vi "ELVIS III v1.0 DO Enqueue Data.vi"(7 "DO Block Channels FPGA Reference":T1, 8 "error in (no error)":errorcluster, 11 "DO Block Write Configuration":T2={"Wait Until Done?"=TRUE, "DO FIFO Clock Divisor"=1000, "Write Mode"=0, "DO (N Samples) Bank Data "=[]}) -> (0 "error out":errorcluster)   [LabVIEW 2021]
uses:
  <vilib>/myRIO/Common/Instrument Driver Framework/ELVIS III v1.0/DO Block/typedefs/ELVIS III DO Block Configuration.ctl
  <vilib>/myRIO/Common/Instrument Driver Framework/ELVIS III v1.0/DO Block/typedefs/ELVIS III DO Block Bank Data.ctl
  <vilib>/myRIO/Common/Instrument Driver Framework/ELVIS III v1.0/DO Block/typedefs/ELVIS III DO Block FPGA Reference.ctl
  <vilib>/rvi/errors/niLvFpgaAdjustHostInterfaceError.vi
  <vilib>/rvi/interface/nirviReadWriteControl/nirviReadWriteControl.xnode
  NiFpgaLv.dll
  <vilib>/rvi/interface/Simulation/niFpgaSimulationCallBeginRW.vi
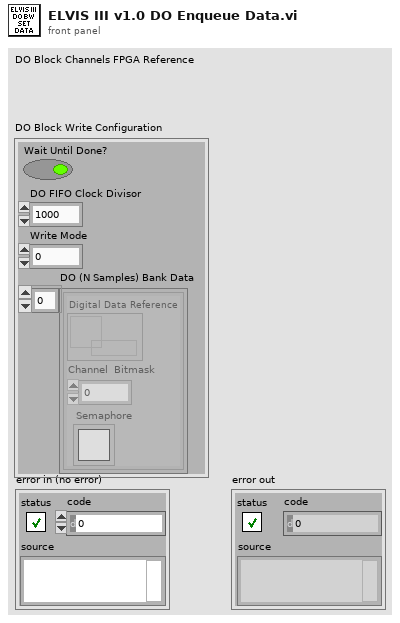
[diagram p1: front panel]
types:
  T1 = typedef "ELVIS III DO Block FPGA Reference.ctl" = refnum<k20>
  T2 = typedef "ELVIS III DO Block Configuration.ctl" = cluster{"Wait Until Done?":bool, "DO FIFO Clock Divisor":u16, "Write Mode":u8, "DO (N Samples) Bank Data ":T3[]}
  T3 = typedef "ELVIS III DO Block Bank Data.ctl" = cluster{"Digital Data Reference":refnum<data-value>, "Channel  Bitmask":fxp<+,20,20>, "Semaphore":T4}
  T4 = typedef "Semaphore RefNum" = refnum<k1>
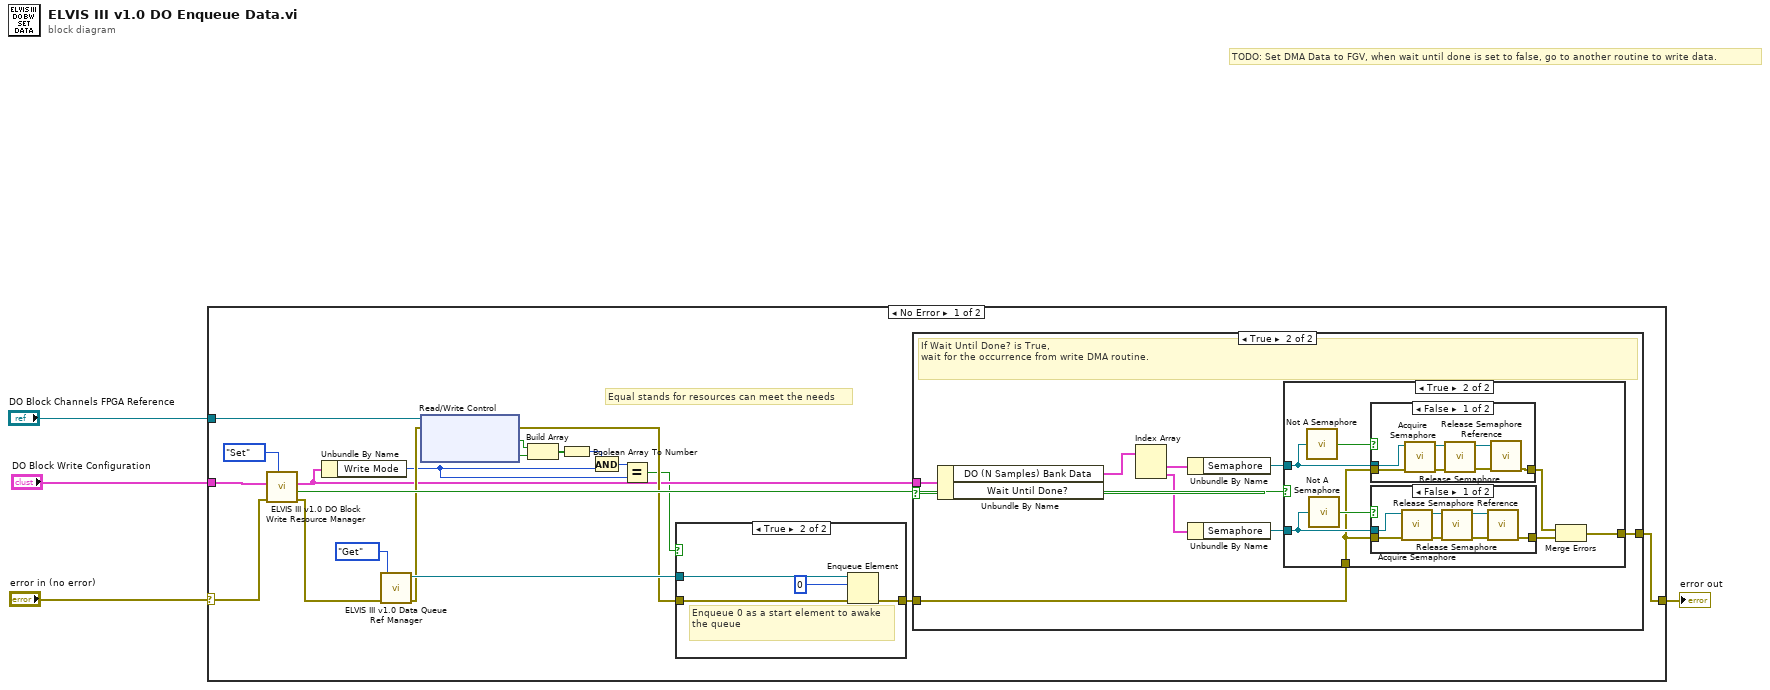
[diagram p0: block diagram]
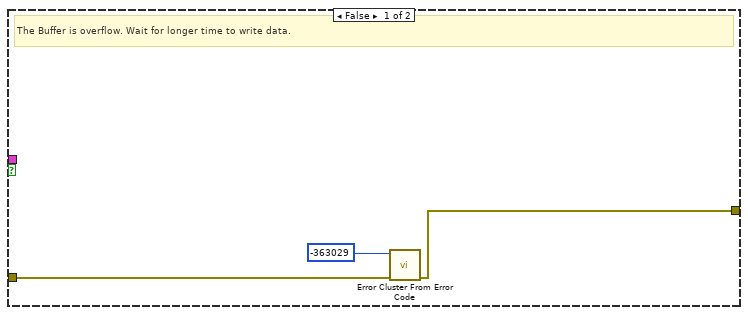
[diagram p3: hidden frame]
diagram:
  # "TODO: Set DMA Data to FGV, when wait until done is set to false, go to another routine to write data."
  n1 = case shown="No Error" "error in (no error)" {
    selector: "error in (no error)" -> [w19 w67]
    tunnel: [w5 w67] -> w3
    tunnel: "DO Block Write Configuration" -> [w23 _]
    tunnel: "DO Block Channels FPGA Reference" -> [w24 _]
    frame No Error {
      # "Equal stands for resources can meet the needs"
      n2 = call <vilib>:"ELVIS III v1.0 DO Block Write Resource Manager.vi"("Action"=enum16{"Set", "Get"}."Set", "error in (no error)"=w19, "DO Resource In"=w23) -> ("error out"=w20:errorcluster, "Action Succeeds"=w21:bool, "DO Resource Out"=w13:T2)  [unwired: 6 in]
      n3 = Unbundle By Name(w13) -> ("Write Mode"=w7:u8)
      n4 = call <vilib>:"ELVIS III v1.0 Data Queue Ref Manager.vi"("Action"=enum16{"Get", "Reset"}."Get", "error in (no error)"=w20) -> ("error out"=w15:errorcluster, "Queue out"=w17:refnum<queue>)  [unwired: 7 in]
      n5 = xnode "Read/Write Control"("FPGA VI Reference In"=w24, "error in"=w15) -> ("error out"=w14:errorcluster, "DO.A.DMA_IDL"=w12:bool, "DO.B.DMA_IDL"=w11:bool)  [unwired: 1 out]
      n6 = Build Array(w12, w11) -> (w10:bool[])
      n7 = Boolean Array To Number(Boolean array=w10) -> (number=w9:u8)
      n8 = And(x=w9, y=w7) -> (x .and. y?=w8:u8)
      n9 = Equal?(x=w8, y=w7) -> (x = y?=w6:bool)
      n10 = case shown="True" w6 {
        tunnel: w17 -> [_ w29]
        tunnel: [w25 w28] -> w22
        tunnel: w14 -> [w25 w27]
        frame False {
        }
        frame True {
          # "Enqueue 0 as a start element to awake the queue"
          n11 = Enqueue Element(queue=w29, element=0, error in (no error)=w27) -> (error out=w28:errorcluster)  [unwired: 1 in, 2 out]
        }
      }
      n12 = case shown="True" w21 {
        tunnel: w22 -> [w31 w34]
        tunnel: w13 -> [_ w40]
        tunnel: [w30 w33] -> w5
        frame False {
          # "The Buffer is overflow. Wait for longer time to write data."
          n13 = call <vilib>:"Error Cluster From Error Code.vi"("error in (no error)"=w31, "error code (0)"=-363029) -> ("error out"=w30:errorcluster)  [unwired: 7 in]
        }
        frame True {
          # "If Wait Until Done? is True, \nwait for the occurrence from write DMA routine."
          n14 = Unbundle By Name(w40) -> ("DO (N Samples) Bank Data"=w39:T3[], "Wait Until Done?"=w41:bool)
          n15 = Index Array(array=w39) -> (element #1=w38:T3, element #2=w36:T3)  [unwired: 2 in]
          n16 = Unbundle By Name(w38) -> ("Semaphore"=w37:T4)
          n17 = Unbundle By Name(w36) -> ("Semaphore"=w35:T4)
          n18 = case shown="True" w41 {
            tunnel: w37 -> [_ w50]
            tunnel: w35 -> [_ w48]
            tunnel: w34 -> [w42 w46]
            tunnel: [w42 w43] -> w33
            frame False {
            }
            frame True {
              n19 = call <vilib>:"Not A Semaphore.vi"("semaphore"=w50) -> ("not a semaphore"=w49:bool)
              n20 = call <vilib>:"Not A Semaphore.vi"("semaphore"=w48) -> ("not a semaphore"=w47:bool)
              n21 = case shown="False" w49 {
                tunnel: w50 -> [w65 _]
                tunnel: w46 -> [w60 w66]
                tunnel: [w59 w66] -> w45
                frame False {
                  n22 = call <vilib>:"Acquire Semaphore.vi"("error in (no error)"=w60, "semaphore"=w65) -> ("error out"=w61:errorcluster, "semaphore out"=w64:T4)  [unwired: 3 in, 1 out]
                  n23 = call <vilib>:"Release Semaphore.vi"("error in (no error)"=w61, "semaphore"=w64) -> ("error out"=w62:errorcluster, "semaphore out"=w63:T4)  [unwired: 4 in]
                  n24 = call <vilib>:"Release Semaphore Reference.vi"("error in (no error)"=w62, "semaphore"=w63) -> ("error out"=w59:errorcluster)  [unwired: 8 in, 1 out]
                }
                frame True {
                }
              }
              n25 = case shown="False" w47 {
                tunnel: w48 -> [w53 _]
                tunnel: w46 -> [w52 w58]
                tunnel: [w51 w58] -> w44
                frame False {
                  n26 = call <vilib>:"Acquire Semaphore.vi"("error in (no error)"=w52, "semaphore"=w53) -> ("error out"=w55:errorcluster, "semaphore out"=w56:T4)  [unwired: 3 in, 1 out]
                  n27 = call <vilib>:"Release Semaphore.vi"("error in (no error)"=w55, "semaphore"=w56) -> ("error out"=w54:errorcluster, "semaphore out"=w57:T4)  [unwired: 4 in]
                  n28 = call <vilib>:"Release Semaphore Reference.vi"("error in (no error)"=w54, "semaphore"=w57) -> ("error out"=w51:errorcluster)  [unwired: 8 in, 1 out]
                }
                frame True {
                }
              }
              n29 = Merge Errors(w45, w44) -> (w43:errorcluster)
            }
          }
        }
      }
    }
    frame Error {
    }
  }
  "error out" <- w3
